vi "degrees_to_dynamixel_units.vi"(10 "MX Motor?":bool, 11 "Degree Input":dbl) -> (2 "Dynamixel units/cycle":dbl, 3 "Dynamixel units":dbl)   [LabVIEW 2013]
doc: "This VI takes in degrees and outputs Dynamixel units. The units are different for the MX and AX, which is controlled by the input boolean."
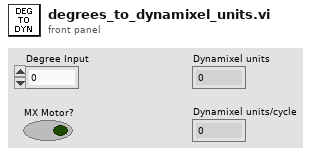
[diagram p1: front panel]
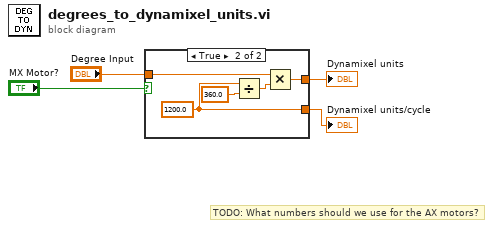
[diagram p0: block diagram]
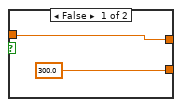
[diagram p2: hidden frame]
diagram:
  # "TODO: What numbers should we use for the AX motors?"
  n1 = case shown="True" "MX Motor?" {
    tunnel: [300.0 ("y") w11] -> w4
    tunnel: "Degree Input" -> [w5 w10]
    tunnel: [w5 w9] -> w2
    frame False {
    }
    frame True {
      w11 = 1200.0 ("y")
      n2 = Divide(x=w11, y=360.0) -> (x/y=w8:dbl)
      n3 = Multiply(x=w10, y=w8) -> (x*y=w9:dbl)
    }
  }
  "Dynamixel units/cycle" <- w4
  "Dynamixel units" <- w2
